vi "Remove Whitespace from VIA.vi"(11 "Pretty Printed VIA":string) -> (3 "Ugly Printed VIA":string)   [LabVIEW 2020, in "PicoG-Core.lvlib"]
uses:
  PicoG-Core/PicoG-Core.lvlib
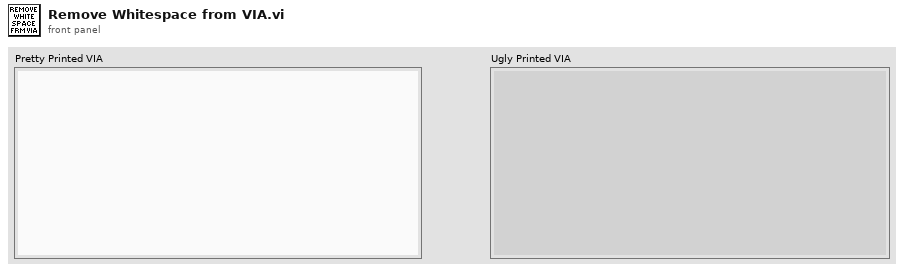
[diagram p1: front panel]
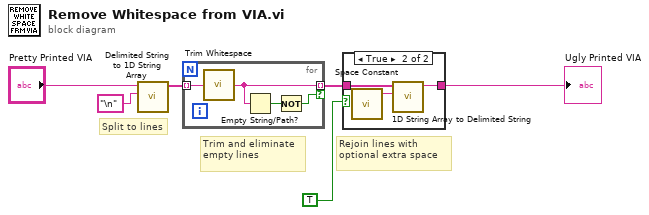
[diagram p0: block diagram]
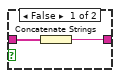
[diagram p2: hidden frame]
diagram:
  # "Rejoin lines with optional extra space"
  # "Trim and eliminate empty lines"
  # "Split to lines"
  n1 = call <vilib>:"Delimited String to 1D String Array.vi"("delimiter"="\n", "delimited string"="Pretty Printed VIA") -> ("string array"=w1:string[])  [unwired: 9 in]
  n2 = for {
    tunnel: w1 -> [w10] mode=indexing
    tunnel: [w9] -> w2 mode=indexing if=w7
    n3 = call <vilib>:"Trim Whitespace.vi"("string"=w10) -> ("trimmed string"=w9:string)  [unwired: 1 in]
    n4 = Empty String/Path?(string/path=w9) -> (empty?=w8:bool)
    n5 = Not(x=w8) -> (.not. x?=w7:bool)
  }
  n6 = case shown="True" TRUE ("Leave Spaces?") {
    tunnel: w2 -> [w12 w15]
    tunnel: [w11 w14] -> w4
    frame False {
      n7 = Concatenate Strings(w12) -> (w11:string)
    }
    frame True {
      n8 = call <vilib>:"Space Constant.vi"() -> ("String"=w13:string)
      n9 = call <vilib>:"1D String Array to Delimited String.vi"("delimiter"=w13, "string array"=w15) -> ("delimited string"=w14:string)  [unwired: 9 in]
    }
  }
  "Ugly Printed VIA" <- w4
